vi "LIA Configure Digital PLL.vi"(6 "pll.m":i8, 7 "index (0)":i32, 8 "error in (no error)":errorcluster, 9 "pll.q":fxp<+,48,0>, 10 "pll.dconfig":T1, 11 "FPGA Session in":refnum<k20>) -> (0 "error out":errorcluster, 3 "FPGA Session out":refnum<k20>)   [LabVIEW 2017]
uses:
  Program Files (x86)/National Instruments/LabVIEW 2017/examples/Lock-In Amplifier/lib/host/Public/fpga type.ctl
  <vilib>/Utility/error.llb/Error Cluster From Error Code.vi
  <vilib>/rvi/errors/niLvFpgaAdjustHostInterfaceError.vi
  <vilib>/rvi/interface/nirviReadWriteControl/nirviReadWriteControl.xnode
  Program Files (x86)/National Instruments/LabVIEW 2017/examples/Lock-In Amplifier/lib/host/Lock-In Amplifier Example Host.lvlib
  NiFpgaLv.dll
  <vilib>/rvi/interface/Simulation/niFpgaSimulationCallBeginRW.vi
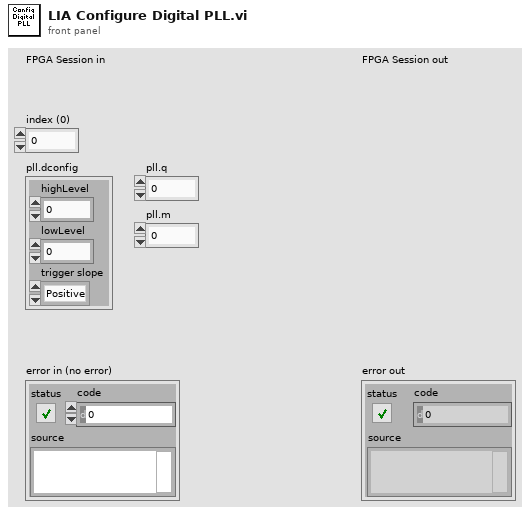
[diagram p1: front panel]
types:
  T1 = cluster{"highLevel":fxp<+/-,18,1>, "lowLevel":fxp<+/-,18,1>, "trigger slope":enum8{"Positive", "Negative"}}
  T2 = typedef "Lock-In Amplifier Example Host.lvlib/fpga type.ctl" = refnum<k20>
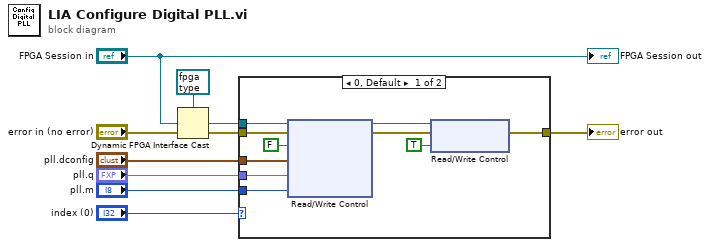
[diagram p0: block diagram]
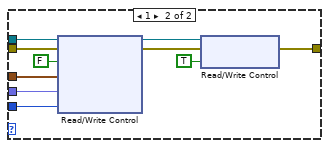
[diagram p2: hidden frame]
diagram:
  n1 = Dynamic FPGA Interface Cast(Session In=T2 refnum ("fpga type"), Type="FPGA Session in") -> (Session Out=w7:T2)
  n2 = case shown="0, Default" "index (0)" {
    tunnel: w7 -> [w19 w29]
    tunnel: "error in (no error)" -> [w18 w28]
    tunnel: [w12 w22] -> w5
    tunnel: "pll.dconfig" -> [w17 w27]
    tunnel: "pll.q" -> [w16 w26]
    tunnel: "pll.m" -> [w15 w25]
    frame 0, Default {
      n3 = xnode "Read/Write Control"("FPGA VI Reference In"=w19, "error in"=w18, "pll.enable 0"=FALSE, "pll.dconfig 0"=w17, "pll.q 0"=w16, "pll.m 0"=w15) -> ("FPGA VI Reference Out"=w14:T2, "error out"=w13:errorcluster)
      n4 = xnode "Read/Write Control"("FPGA VI Reference In"=w14, "error in"=w13, "pll.enable 0"=TRUE) -> ("error out"=w12:errorcluster)  [unwired: 1 out]
    }
    frame 1 {
      n5 = xnode "Read/Write Control"("FPGA VI Reference In"=w29, "error in"=w28, "pll.enable 1"=FALSE ("pll.enable 0"), "pll.dconfig 1"=w27, "pll.q 1"=w26, "pll.m 1"=w25) -> ("FPGA VI Reference Out"=w24:T2, "error out"=w23:errorcluster)
      n6 = xnode "Read/Write Control"("FPGA VI Reference In"=w24, "error in"=w23, "pll.enable 1"=TRUE ("pll.enable 0")) -> ("error out"=w22:errorcluster)  [unwired: 1 out]
    }
  }
  "error out" <- w5
  "FPGA Session out" <- "FPGA Session in"
